vi "Generate TO event.vi"(9 "Boolean":bool, 10 "message":string, 11 "User Event in":refnum<user-event>) -> ()   [LabVIEW 2011]
uses:
  DecisionCluster_typdef.ctl
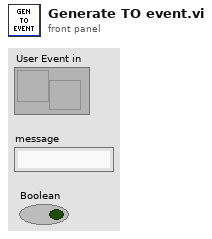
[diagram p1: front panel]
types:
  T1 = typedef "DecisionCluster_typdef.ctl" = cluster{"vi path":path, "Message":string}
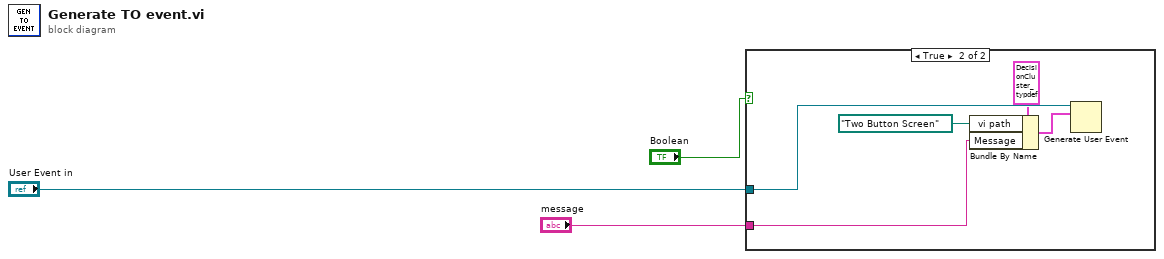
[diagram p0: block diagram]
diagram:
  n1 = case shown="True" "Boolean" {
    tunnel: "User Event in" -> [_ w8]
    tunnel: "message" -> [_ w4]
    frame False {
    }
    frame True {
      n2 = Bundle By Name(cluster=T1 {"vi path"=path "Dummy.vi", "Message"=""}, "vi path"=path "Two Button Screen" ("event data"), "Message"=w4) -> (w5:T1)
      n3 = Generate User Event(user event=w8, event data cluster=w5) -> ()  [unwired: 1 in, 2 out]
    }
  }
